vi "Get Cursor Position.vi"(8 "error in (no error)":errorcluster, 10 "Cursor":T1, 11 "MSOX6004 in":refnum<class "MSOX6004.lvclass">) -> (0 "error out":errorcluster, 2 "Position":dbl format="%.9f", 3 "MSOX6004 out":refnum<class "MSOX6004.lvclass">)   [LabVIEW 2018, in "MSOX6004.lvlib" / "MSOX6004.lvclass"]
doc: "This Override method is used to get cursor(s) position from the Oscope instrument. Use 'Cursor' control to select the cursor of interest, and carry out its value to the 'Position' indicator."
uses:
  MSOX6004.lvclass
  PPLs/Oscilloscope/Parent/Oscilloscope.lvlibp/Custom Controls/Select Cursor.ctl
  PPLs/Oscilloscope/Parent/Oscilloscope.lvlibp
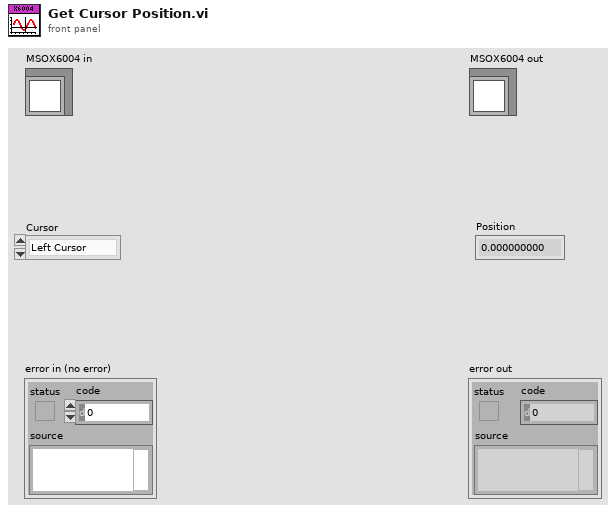
[diagram p1: front panel]
types:
  T1 = typedef "Oscilloscope.lvlibp/Select Cursor.ctl" = enum16{"Left Cursor", "Right Cursor", "Top Cursor", "Bottom Cursor"}
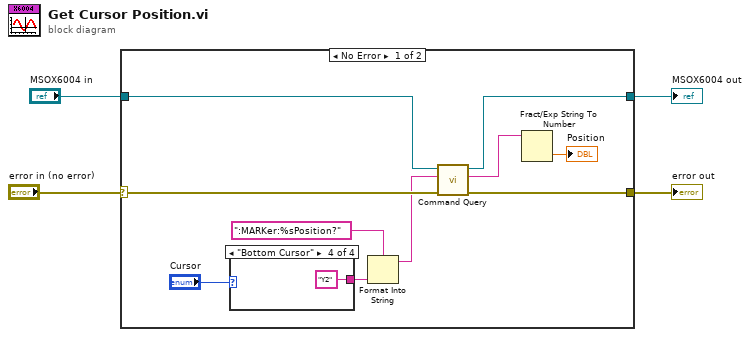
[diagram p0: block diagram]
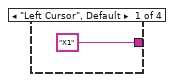
[diagram p2: hidden frame]
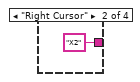
[diagram p3: hidden frame]
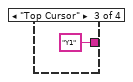
[diagram p4: hidden frame]
diagram:
  n1 = case shown="No Error" "error in (no error)" {
    selector: "error in (no error)" -> [w14 w20]
    tunnel: [w11 w20] -> w3
    tunnel: [w12 w19] -> w2
    tunnel: "MSOX6004 in" -> [w13 w19]
    frame No Error {
      n2 = case shown="\"Bottom Cursor\"" "Cursor" {
        tunnel: ["X1" "X2" "Y1" "Y2"] -> w8
        frame "Left Cursor", Default {
        }
        frame "Right Cursor" {
        }
        frame "Top Cursor" {
        }
        frame "Bottom Cursor" {
        }
      }
      n3 = Format Into String(format string=":MARKer:%sPosition?", w8) -> (resulting string=w7:string)  [unwired: 2 in, 1 out]
      n4 = call "Command Query.vi"("error in (no error)"=w14, "Command"=w7, "MSOX6004 in"=w13) -> ("error out"=w11:errorcluster, "Response"=w6:string, "MSOX6004 out"=w12:refnum<class "MSOX6004.lvclass">)  [unwired: 6 in]
      n5 = Fract/Exp String To Number(string=w6) -> (number=→"Position":dbl)  [unwired: 3 in, 1 out]
    }
    frame Error {
    }
  }
  "error out" <- w3
  "MSOX6004 out" <- w2
